vi "Read Write Signals.vi"(8 "error in (no error)":errorcluster, 9 "Digital Outputs":T1, 10 "Analog Outputs":T2, 11 "PXI in":refnum<class "PXI.lvclass">) -> (0 "error out":errorcluster, 1 "Digital Inputs":T1, 2 "Analog Inputs":T2, 3 "PXI out":refnum<class "PXI.lvclass">)   [LabVIEW 2013, in "PXI.lvclass"]
uses:
  PXI.lvclass
  controls/Analog Values.ctl
  controls/Digital Values.ctl
  PXI.lvclass/PXI.ctl
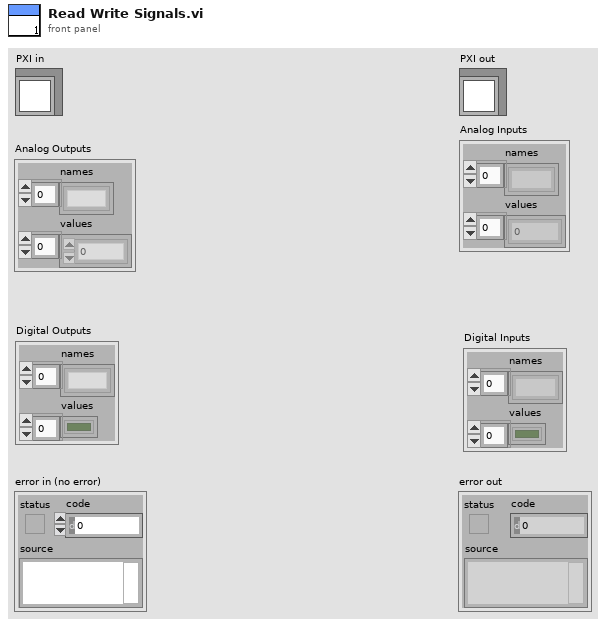
[diagram p1: front panel]
types:
  T1 = typedef "Digital Values.ctl" = cluster{"names":string[], "values":bool[]}
  T2 = typedef "Analog Values.ctl" = cluster{"names":string[], "values":dbl[]}
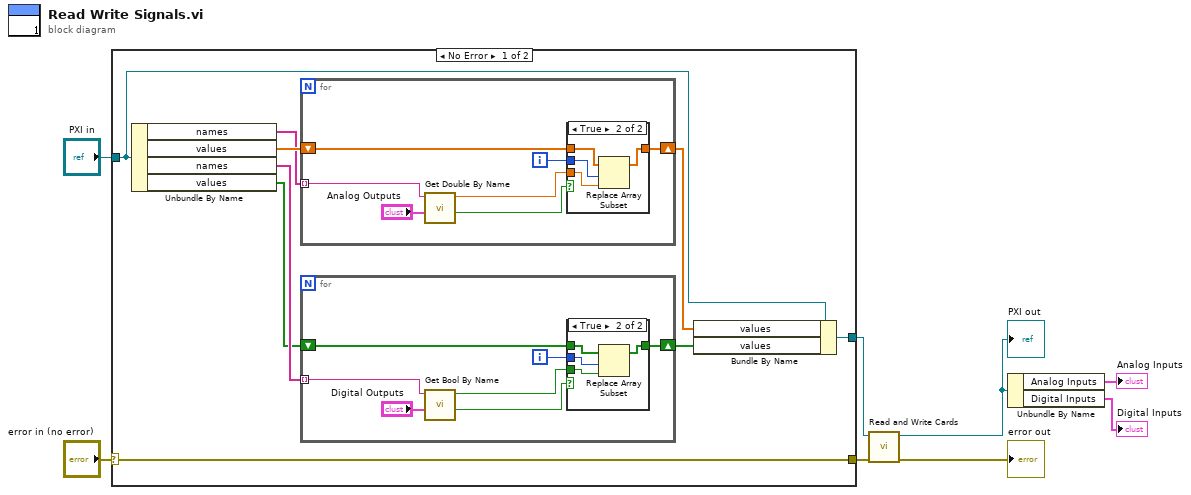
[diagram p0: block diagram]
diagram:
  n1 = case shown="No Error" "error in (no error)" {
    selector: "error in (no error)" -> [w17 w43]
    tunnel: [w17 w43] -> w5
    tunnel: [w9 w42] -> w6
    tunnel: "PXI in" -> [w12 w42]
    frame No Error {
      n2 = Unbundle By Name(w12) -> ("names"=w13:string[], "values"=w14:dbl[], "names"=w16:string[], "values"=w15:bool[])
      n3 = for {
        tunnel: w13 -> [w34] mode=indexing
        shift-right: [w36] -> w10
        shift-left: w14 -> [w33]
        i -> [w32]
        n4 = call "Get Double By Name.vi"("name"=w34, "Analog Values"="Analog Outputs") -> ("result"=w30:dbl, "found?"=w31:bool)  [unwired: 7 in]
        n5 = case shown="True" w31 {
          tunnel: [w37 w41] -> w36
          tunnel: w33 -> [w37 w40]
          tunnel: w32 -> [_ w39]
          tunnel: w30 -> [_ w38]
          frame False {
          }
          frame True {
            n6 = Replace Array Subset(array=w40, new element=w38, index=w39) -> (w41:dbl[])
          }
        }
      }
      n7 = for {
        tunnel: w16 -> [w24] mode=indexing
        shift-right: [w18] -> w11
        shift-left: w15 -> [w20]
        i -> [w19]
        n8 = call "Get Bool By Name.vi"("name"=w24, "Digital Values"="Digital Outputs") -> ("result"=w21:bool, "found?"=w22:bool)  [unwired: 7 in]
        n9 = case shown="True" w22 {
          tunnel: [w25 w29] -> w18
          tunnel: w21 -> [_ w26]
          tunnel: w19 -> [_ w28]
          tunnel: w20 -> [w25 w27]
          frame False {
          }
          frame True {
            n10 = Replace Array Subset(array=w27, new element=w26, index=w28) -> (w29:bool[])
          }
        }
      }
      n11 = Bundle By Name(cluster=w12, "values"=w10, "values"=w11) -> (w9:refnum<class "PXI.lvclass">)
    }
    frame Error {
    }
  }
  n12 = call "Read and Write Cards.vi"("error in (no error)"=w5, "PXI in"=w6) -> ("error out"=→"error out":errorcluster, "PXI out"=w3:refnum<class "PXI.lvclass">)  [unwired: 8 in]
  "PXI out" <- w3
  n13 = Unbundle By Name(w3) -> ("Analog Inputs"=→"Analog Inputs":T2, "Digital Inputs"=→"Digital Inputs":T1)
